vi "Read c header file string.vi"(8 "error in":errorcluster, 11 "Shared Memory configuration in":refnum<class "Shared Memory configuration.lvclass">) -> (0 "error out":errorcluster, 2 "c header file string":string, 3 "Shared Memory configuration out":refnum<class "Shared Memory configuration.lvclass">)   [LabVIEW 2013, in "Shared Memory configuration.lvclass"]
uses:
  Shared Memory configuration.lvclass
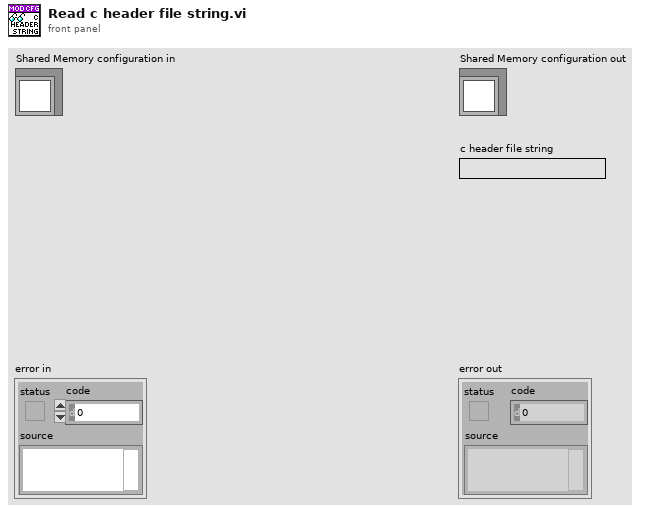
[diagram p1: front panel]
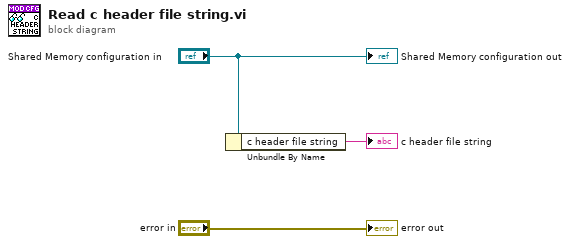
[diagram p0: block diagram]
diagram:
  n1 = Unbundle By Name("Shared Memory configuration in") -> ("c header file string"=→"c header file string":string)
  "error out" <- "error in"
  "Shared Memory configuration out" <- "Shared Memory configuration in"
